vi "Copy Header.vi"(6 "GUID":string, 8 "error in (no error)":errorcluster, 11 "Linked List Header in":refnum<class "Linked List Header.lvclass">) -> (0 "error out":errorcluster, 3 "Linked List Header out":refnum<class "Linked List Header.lvclass">)   [LabVIEW 2020, in "Linked Lists.lvlib" / "Linked List Header.lvclass"]
uses:
  <vilib>/gpm_packages/@cs/linked-list/Source/Linked List/Linked List Header/Linked List Header.lvclass
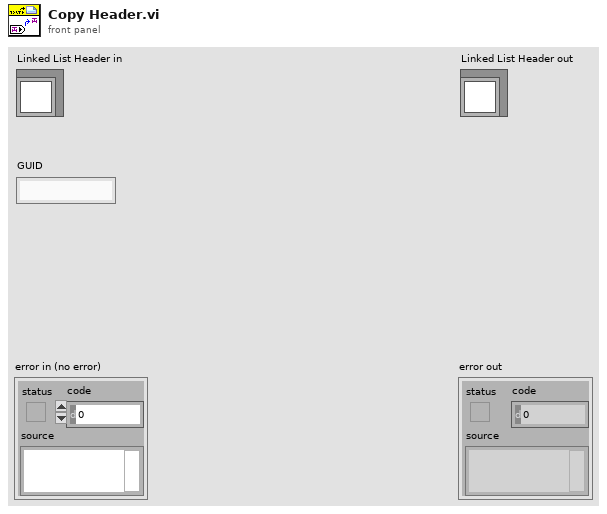
[diagram p1: front panel]
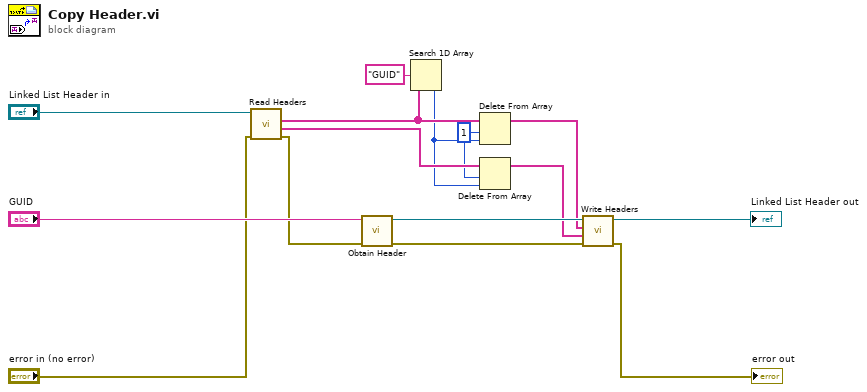
[diagram p0: block diagram]
diagram:
  w9 = 1 ("length")
  n1 = call <vilib>:"Read Headers.vi"("error in (no error)"="error in (no error)", "Linked List Header in"="Linked List Header in") -> ("error out"=w5:errorcluster, "Header Values"=w11:string[], "Header Names"=w12:string[])  [unwired: 5 in, 2 out]
  n2 = call <vilib>:"Obtain Header.vi"("error in (no error)"=w5, "GUID"="GUID") -> ("error out"=w4:errorcluster, "Linked List Header out"=w8:refnum<class "Linked List Header.lvclass">)  [unwired: 8 in]
  n3 = Search 1D Array(1D array=w12, element="GUID" ("Item Name")) -> (index of element=w10:i32)  [unwired: 1 in]
  n4 = Delete From Array(array=w12, length=w9, index=w10) -> (array with subset deleted=w7:string[])  [unwired: 1 out]
  n5 = Delete From Array(array=w11, length=w9, index=w10) -> (array with subset deleted=w6:string[])  [unwired: 1 out]
  n6 = call <vilib>:"Write Headers.vi"("error in (no error)"=w4, "Header Values"=w6, "Header Names"=w7, "Linked List Header in"=w8) -> ("error out"=→"error out":errorcluster, "Linked List Header out"=→"Linked List Header out":refnum<class "Linked List Header.lvclass">)  [unwired: 6 in]
